vi "CPPpuffLoop.vi"() -> ()   [LabVIEW 2022 SP3]
uses:
  Globals/Meas_global.vi
panel:
  in  "Leave Air On?":bool
  in  "Iterate?":bool
  in  "Dur Index":i32
  in  "Sep Index":i32
  in  "Reset iterations?":bool
  in  "#Pulse Index":i32
  in  "#Pulses":i32[](array[numeric])
  in  "Pulse Dur[ms]":dbl[](array[numeric])
  in  "Pulse Sep[ms]":dbl[](array[numeric])
  in  "Pulses":i32
  in  "Low":dbl=20000.0
  in  "MeasTime":dbl=50000.0
  out "PostPurge":dbl=25000.0
  in  "PulseGasChannel":i32=2
  in  "PurgeGasChannel":i32=1
  in  "WebPowerSwitch":string="10.245.69.7"
  in  "PrePurge":dbl=5000.0
  in  "High":dbl=20000.0
  # "Trivial VI to pulse a pair of valves connected\nto a Web Power Switch, for FID response\ntesting                          TCRL 20210715"
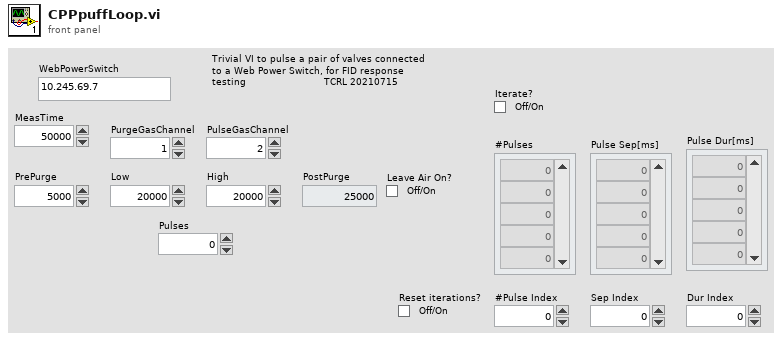
[diagram p1: front panel]
types:
  T1 = typedef "Post_Process.ctl" = enum16{"Take New Data", "Post Process Raw Data File"}
  T2 = typedef "Setup.ctl" = enum16{"Run Program", "Show Setup", "Save Current Setup", "Setup Front Panel"}
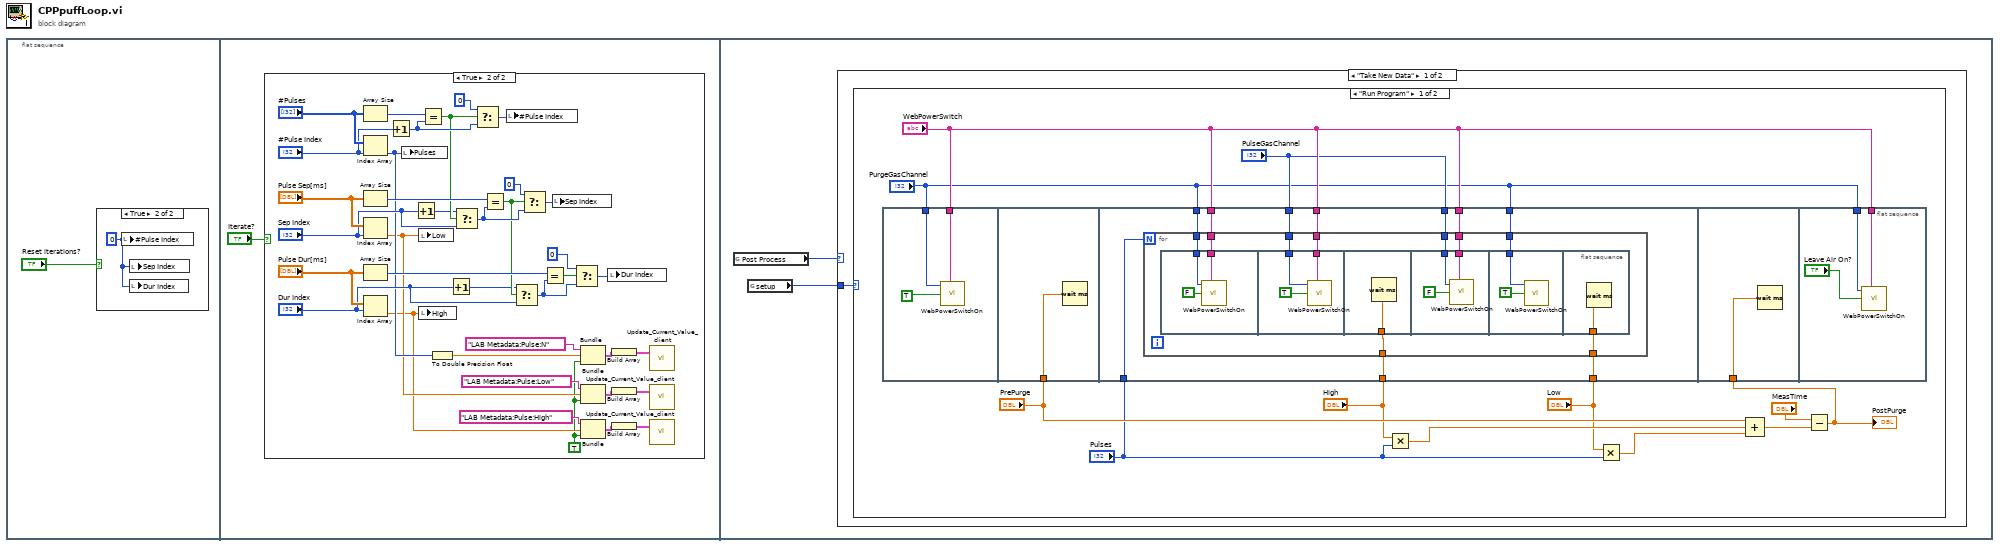
[diagram p0: block diagram]
diagram:
  n1 = flat-sequence {
    frame #0 {
      n2 = case shown="True" "Reset iterations?" {
        frame False {
        }
        frame True {
          w2 = 0 ("Pulse index")
          n3 = local write "#Pulse Index"(w2) -> ()
          n4 = local write "Sep Index"(w2) -> ()
          n5 = local write "Dur Index"(w2) -> ()
        }
      }
    }
    frame #1 {
      n6 = case shown="True" "Iterate?" {
        frame False {
        }
        frame True {
          w4 = TRUE
          n7 = Array Size(array="#Pulses") -> (size(s)=w37:i32)
          n8 = Index Array(array="#Pulses", index="#Pulse Index") -> (element=w10:i32)
          n9 = Array Size(array="Pulse Sep[ms]") -> (size(s)=w33:i32)
          n10 = Index Array(array="Pulse Sep[ms]", index="Sep Index") -> (element=w9:dbl)
          n11 = Array Size(array="Pulse Dur[ms]") -> (size(s)=w31:i32)
          n12 = Index Array(array="Pulse Dur[ms]", index="Dur Index") -> (element=w8:dbl)
          n13 = Increment(x="#Pulse Index") -> (x+1=w38:i32)
          n14 = local write "Pulses"(w10) -> ()
          n15 = Increment(x="Sep Index") -> (x+1=w29:i32)
          n16 = local write "Low"(w9) -> ()
          n17 = local write "High"(w8) -> ()
          n18 = Equal?(x=w37, y=w38) -> (x = y?=w30:bool)
          n19 = To Double Precision Float(number=w10) -> (double precision float=w17:dbl)
          n20 = Increment(x="Dur Index") -> (x+1=w23:i32)
          n21 = Select(t=w29, s=w30, f="Sep Index") -> (s? t:f=w27:i32)
          n22 = Select(t=0, s=w30, f=w38) -> (s? t:f=w39:i32)
          n23 = Equal?(x=w33, y=w27) -> (x = y?=w24:bool)
          n24 = local write "#Pulse Index"(w39) -> ()
          n25 = Select(t=w23, s=w24, f="Dur Index") -> (s? t:f=w19:i32)
          n26 = Select(t=0, s=w24, f=w27) -> (s? t:f=w25:i32)
          n27 = Equal?(x=w31, y=w19) -> (x = y?=w20:bool)
          n28 = local write "Sep Index"(w25) -> ()
          n29 = Select(t=0, s=w20, f=w19) -> (s? t:f=w21:i32)
          n30 = Bundle("LAB Metadata:Pulse:N", w17, w4) -> (w16:cluster{string, dbl, bool})  [unwired: 1 in]
          n31 = Bundle("LAB Metadata:Pulse:Low", "Numeric"=w9, w4) -> (w13:cluster{string, "Numeric":dbl, bool})  [unwired: 1 in]
          n32 = Bundle("LAB Metadata:Pulse:High", "Numeric"=w8, w4) -> (w15:cluster{string, "Numeric":dbl, bool})  [unwired: 1 in]
          n33 = local write "Dur Index"(w21) -> ()
          n34 = Build Array(w16) -> (w5:cluster{string, dbl, bool}[])
          n35 = Build Array(w13) -> (w6:cluster{string, "Numeric":dbl, bool}[])
          n36 = Build Array(w15) -> (w7:cluster{string, "Numeric":dbl, bool}[])
          n37 = call "Update_Current_Value_client.vi"("Update array in"=w5) -> ()  [unwired: 1 in]
          n38 = call "Update_Current_Value_client.vi"("Update array in"=w6) -> ()  [unwired: 1 in]
          n39 = call "Update_Current_Value_client.vi"("Update array in"=w7) -> ()  [unwired: 1 in]
        }
      }
    }
    frame #2 {
      n40 = global read "Meas_global.vi" "Post Process"() -> (w41:T1)
      n41 = global read "Meas_global.vi" "setup"() -> (w42:T2)
      n42 = case shown="\"Take New Data\"" w41 {
        tunnel: w42 -> [w43 _]
        frame "Take New Data" {
          n43 = case shown="\"Run Program\"" w43 {
            frame "Run Program" {
              n44 = flat-sequence {
                tunnel: "PurgeGasChannel" -> [w58]
                tunnel: "WebPowerSwitch" -> [w57]
                tunnel: "PrePurge" -> [w59]
                tunnel: "High" -> [w62]
                tunnel: "PurgeGasChannel" -> [w69]
                tunnel: "WebPowerSwitch" -> [w68]
                tunnel: "PulseGasChannel" -> [w67]
                tunnel: "PulseGasChannel" -> [w66]
                tunnel: "WebPowerSwitch" -> [w65]
                tunnel: "WebPowerSwitch" -> [w64]
                tunnel: "PurgeGasChannel" -> [w63]
                tunnel: "Low" -> [w61]
                tunnel: "Pulses" -> [w60]
                tunnel: w47 -> [w92]
                tunnel: "WebPowerSwitch" -> [w94]
                tunnel: "PurgeGasChannel" -> [w93]
                frame #0 {
                  n45 = call "WebPowerSwitchOn.vi"("WebPowerSwitchOutlet"=w58, "WebPowerSwitchIP"=w57, "DesiredState"=TRUE) -> ()  [unwired: 3 in, 2 out]
                }
                frame #1 {
                  n46 = Wait (ms)(milliseconds to wait=w59) -> ()  [unwired: 1 out]
                }
                frame #2 {
                  n47 = for {
                    N: w60 -> [_]
                    tunnel: w69 -> [w78]
                    tunnel: w68 -> [w77]
                    tunnel: w67 -> [w76]
                    tunnel: w66 -> [w75]
                    tunnel: w65 -> [w74]
                    tunnel: w64 -> [w73]
                    tunnel: w63 -> [w72]
                    tunnel: w62 -> [w71]
                    tunnel: w61 -> [w70]
                    n48 = flat-sequence {
                      tunnel: w77 -> [w81]
                      tunnel: w78 -> [w80]
                      tunnel: w74 -> [w83]
                      tunnel: w76 -> [w82]
                      tunnel: w71 -> [w85]
                      tunnel: w73 -> [w87]
                      tunnel: w75 -> [w86]
                      tunnel: w72 -> [w89]
                      tunnel: w70 -> [w91]
                      frame #0 {
                        n49 = call "WebPowerSwitchOn.vi"("WebPowerSwitchOutlet"=w80, "WebPowerSwitchIP"=w81, "DesiredState"=FALSE) -> ()  [unwired: 3 in, 2 out]
                      }
                      frame #1 {
                        n50 = call "WebPowerSwitchOn.vi"("WebPowerSwitchOutlet"=w82, "WebPowerSwitchIP"=w83, "DesiredState"=TRUE) -> ()  [unwired: 3 in, 2 out]
                      }
                      frame #2 {
                        n51 = Wait (ms)(milliseconds to wait=w85) -> ()  [unwired: 1 out]
                      }
                      frame #3 {
                        n52 = call "WebPowerSwitchOn.vi"("WebPowerSwitchOutlet"=w86, "WebPowerSwitchIP"=w87, "DesiredState"=FALSE) -> ()  [unwired: 3 in, 2 out]
                      }
                      frame #4 {
                        n53 = call "WebPowerSwitchOn.vi"("WebPowerSwitchOutlet"=w89, "DesiredState"=TRUE) -> ()  [unwired: 4 in, 2 out]
                      }
                      frame #5 {
                        n54 = Wait (ms)(milliseconds to wait=w91) -> ()  [unwired: 1 out]
                      }
                    }
                  }
                }
                frame #3 {
                  n55 = Wait (ms)(milliseconds to wait=w92) -> ()  [unwired: 1 out]
                }
                frame #4 {
                  n56 = call "WebPowerSwitchOn.vi"("WebPowerSwitchOutlet"=w93, "WebPowerSwitchIP"=w94, "DesiredState"="Leave Air On?") -> ()  [unwired: 3 in, 2 out]
                }
              }
              n57 = Multiply(x="High", y="Pulses") -> (x*y=w52:dbl)
              n58 = Multiply(x="Low", y="Pulses") -> (x*y=w51:dbl)
              n59 = Compound Arithmetic op=ADD("PrePurge", w52, w51) -> (w48:dbl)
              n60 = Subtract(x="MeasTime", y=w48) -> (x-y=w47:dbl)
              "PostPurge" <- w47
            }
            frame "Show Setup", Default {
            }
          }
        }
        frame "Post Process Raw Data File", Default {
        }
      }
    }
  }
